vi "String coordinate to array data needed.vi"(1 "Input string":string, 2 "Number of coordinates to extract":i32, 3 "Array":dbl[][](array[numeric])) -> (0 "Array of element extracted\nfrom the data array depending \non the coordinates given":dbl[](array[numeric]))   [LabVIEW 2021]
panel:
  out "i":i32
  out "index row":u8
  out "index col":u8
  out "Array of coordinates extracted":u8[](array[numeric])
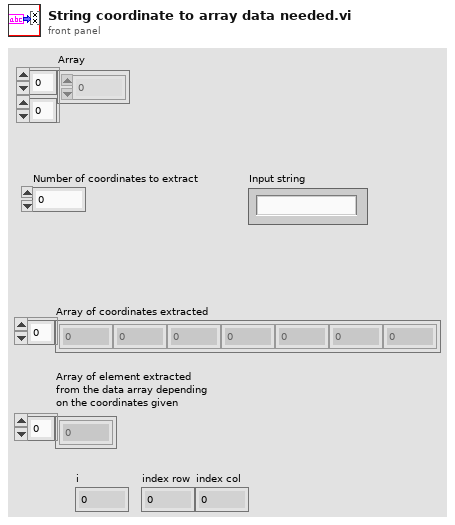
[diagram p1: front panel]
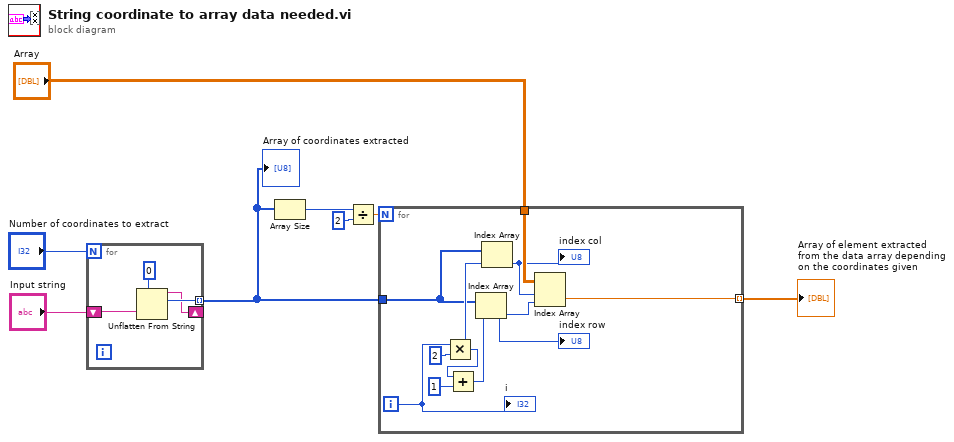
[diagram p0: block diagram]
diagram:
  n1 = for {
    N: "Number of coordinates to extract" -> [_]
    tunnel: [w10] -> w6 mode=indexing
    shift-right: [w9] -> _
    shift-left: "Input string" -> [w11]
    n2 = Unflatten From String(type=u8 0, binary string=w11) -> (rest of the binary string=w9:string, value=w10:u8)  [unwired: 3 in, 1 out]
  }
  "Array of coordinates extracted" <- w6
  n3 = Array Size(array=w6) -> (size(s)=w5:i32)
  n4 = Divide(x=w5, y=2) -> (x/y=w3:dbl)
  n5 = for {
    N: w3 -> [_]
    tunnel: w6 -> [w18]
    tunnel: "Array" -> [w16]
    tunnel: [w15] -> w2 mode=indexing
    i -> [w17]
    n6 = Multiply(x=w17, y=2) -> (x*y=w19:i32)
    n7 = Add(x=w19, y=1) -> (x+y=w20:i32)
    n8 = Index Array(array=w18, index=w20) -> (element=w13:u8)
    "index row" <- w13
    n9 = Index Array(array=w18, index=w19) -> (element=w14:u8)
    "index col" <- w14
    n10 = Index Array(array=w16, index (row)=w14, index (col)=w13) -> (element=w15:dbl)
    "i" <- w17
  }
  "Array of element extracted\nfrom the data array depending \non the coordinates given" <- w2
